vi "Lockin.DAQ.setSampling.vi"(4 "Decimation":i32, 6 "AI Buffer Size (S)":i32=100, 8 "error in (no error)":errorcluster, 9 "Sample Mode":T1=10178 items=["Finite Samples"=10178, "Continuous Samples"=10123], 10 "Sampling":T2={"Fs"=204789.0, "#s"=15753}, 11 "Lockin.DAQ":refnum<class "Lockin.DAQ.lvclass">) -> (0 "error out":errorcluster, 3 "Lockin.DAQ out":refnum<class "Lockin.DAQ.lvclass">)   [LabVIEW 2016, in "Lockin.DAQ.lvclass"]
doc: "---------------------------------------------------------------\nJKI State Machine Objects™\nhttp://jki.net/state-machine-objects/\nCopyright (C) 2005-2015, JKI <info@jki.net>\nALL RIGHTS RESERVEDJKI State Machine Objects (SMO) 1.0.0.4\nJKI - JKI\nCopyright (c) 2015, JKI"
uses:
  Lockin.DAQ.lvclass
  Typedefs/Sampling.ctl
  Typedefs/Sample Mode--Ring.ctl
  Typedefs/PrivateEvents--Lockin.DAQ.setSampling.ctl
  Lockin.DAQ.lvclass/Lockin.DAQ.ctl
panel:
  # "For instructions on how to use the JKI State Machine Objects, examples and video tutorials, visit:\nhttp://jki.net/state-machine-objects/\n\nJKI State Machine Objects™\nhttp://jki.net/state-machine-objects/\nCopyright (C) 2005-2015, JKI <info@jki.net>\nALL RIGHTS RESERVED"
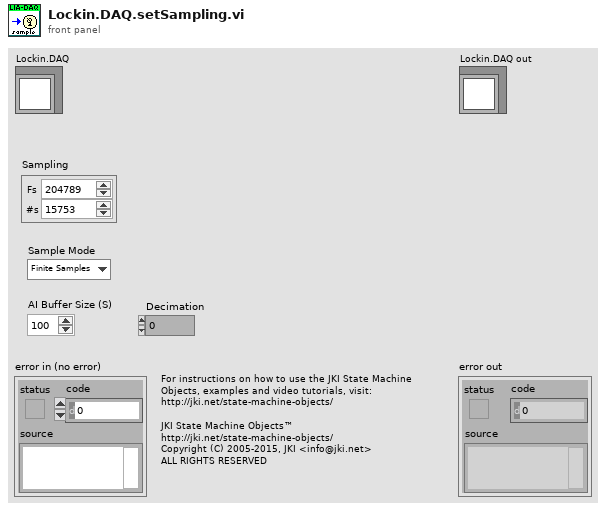
[diagram p1: front panel]
types:
  T1 = typedef "Lockin.DAQ.lvclass/Sample Mode--Ring.ctl" = i32
  T2 = typedef "Lockin.DAQ.lvclass/Sampling.ctl" = cluster{"Fs":dbl, "#s":i32}
  T3 = typedef "Lockin.DAQ.lvclass/PrivateEvents--Lockin.DAQ.setSampling.ctl" = cluster{"Sampling":T2, "Sample Mode":T1, "AI Buffer Size (S)":i32, "Decimation":i32}
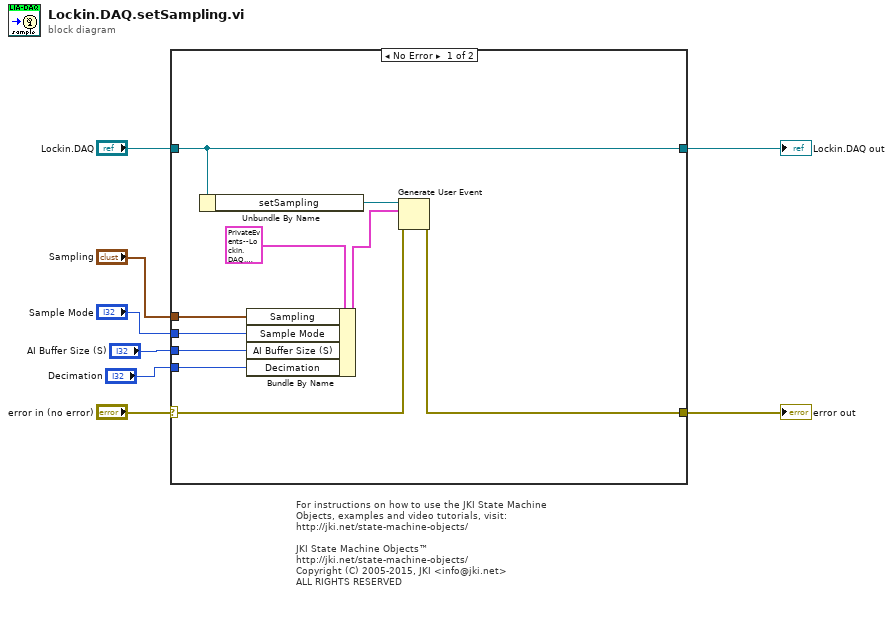
[diagram p0: block diagram]
diagram:
  # "For instructions on how to use the JKI State Machine Objects, examples and video tutorials, visit:\nhttp://jki.net/state-machine-objects/\n\nJKI State Machine Objects™\nhttp://jki.net/state-machine-objects/\nCopyright (C) 2005-2015, JKI <info@jki.net>\nALL RIGHTS RESERVED"
  n1 = case shown="No Error" "error in (no error)" {
    selector: "error in (no error)" -> [w18 w20]
    tunnel: [w16 w20] -> w7
    tunnel: [w15 w19] -> w8
    tunnel: "Lockin.DAQ" -> [w15 w19]
    tunnel: "Sampling" -> [w12 _]
    tunnel: "Sample Mode" -> [w11 _]
    tunnel: "AI Buffer Size (S)" -> [w10 _]
    tunnel: "Decimation" -> [w9 _]
    frame No Error {
      n2 = Unbundle By Name(w15) -> ("setSampling"=w17:refnum<user-event>)
      n3 = Bundle By Name(cluster=T3 {"Sampling"={"Fs"=204789.0, "#s"=15753}, "Sample Mode"=10178, "AI Buffer Size (S)"=100, "Decimation"=100} ("setSampling"), "Sampling"=w12, "Sample Mode"=w11, "AI Buffer Size (S)"=w10, "Decimation"=w9) -> (w13:T3)
      n4 = Generate User Event(user event=w17, event data cluster=w13, error in=w18) -> (error out=w16:errorcluster)  [unwired: 1 in, 1 out]
    }
    frame Error {
    }
  }
  "error out" <- w7
  "Lockin.DAQ out" <- w8
